vi "2D_Data_to_Igor_with_Prefix.vi"(6 "Do Transfer":bool=TRUE, 8 "error in (no error)":errorcluster, 9 "Wave Name":string, 10 "Wave Prefix":string, 11 "Data":dbl[][](array[numeric]) format="%.2f") -> (0 "error out":errorcluster, 2 "Wave Prefix Through":string)   [LabVIEW 2010]
uses:
  <vilib>/Utility/file.llb/Write To Spreadsheet File (DBL).vi
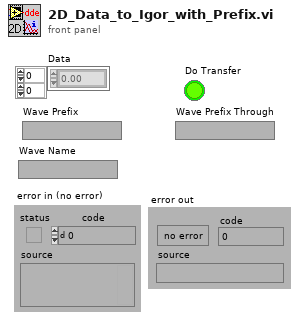
[diagram p1: front panel]
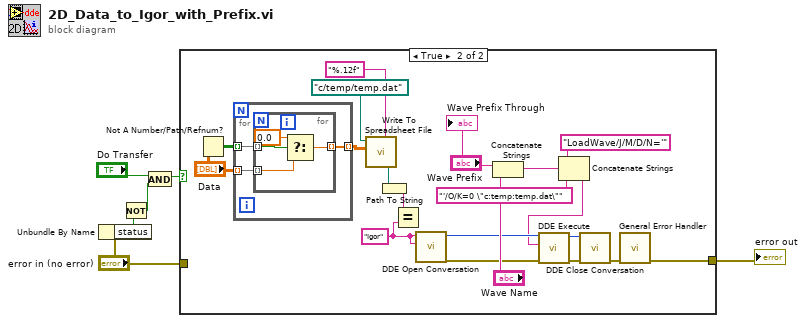
[diagram p0: block diagram]
diagram:
  n1 = Unbundle By Name("error in (no error)") -> ("status"=w4:bool)
  n2 = Not(x=w4) -> (.not. x?=w3:bool)
  n3 = And(x="Do Transfer", y=w3) -> (x .and. y?=w2:bool)
  n4 = case shown="True" w2 {
    tunnel: [w7 w25] -> w6
    tunnel: "error in (no error)" -> [w7 _]
    frame False {
    }
    frame True {
      w11 = "Igor" ("service")
      n5 = Not A Number/Path/Refnum?(number/path/refnum="Data") -> (NaN/Path/Refnum?=w26:bool[][])
      n6 = for {
        tunnel: w26 -> [w30] mode=indexing
        tunnel: "Data" -> [w29] mode=indexing
        tunnel: [w28] -> w13 mode=indexing
        n7 = for {
          tunnel: w30 -> [w34] mode=indexing
          tunnel: w29 -> [w33] mode=indexing
          tunnel: [w31] -> w28 mode=indexing
          n8 = Select(t=0.0, s=w34, f=w33) -> (s? t:f=w31:dbl)
        }
      }
      n9 = call-poly <vilib>:"Write To Spreadsheet File.vi"("format (%.3f)"="%.12f", "2D data"=w13, "file path (dialog if empty)"=path "c:/temp/temp.dat" ("Path")) -> ("new file path (Not A Path if cancelled)"=w10:path)  [unwired: 5 in]
      n10 = Path To String(path=w10) -> (string=w9:string)
      n11 = Equal?(x=w9, y=w11) -> ()  [unwired: 1 out]
      n12 = call "DDE Open Conversation.vi"("topic"=w11, "service"=w11) -> ("error out"=w19:errorcluster, "conversation refnum"=w22:u32)  [unwired: 6 in]
      n13 = Concatenate Strings("Wave Prefix", "Wave Name") -> (w17:string)
      n14 = Concatenate Strings("LoadWave/J/M/D/N='" ("command"), w17, "'/O/K=0 \"c:temp:temp.dat\"" ("command")) -> (w16:string)
      n15 = call <vilib>:"DDE Execute.vi"("error in (no error)"=w19, "command"=w16, "conversation refnum in"=w22) -> ("error out"=w20:errorcluster, "conversation refnum out"=w21:u32)  [unwired: 5 in]
      n16 = call "DDE Close Conversation.vi"("error in (no error)"=w20, "conversation refnum"=w21) -> ("error out"=w27:errorcluster)  [unwired: 7 in]
      n17 = call <vilib>:"General Error Handler.vi"("error in (no error)"=w27) -> ("error out"=w25:errorcluster)  [unwired: 10 in, 4 out]
      "Wave Prefix Through" <- "Wave Prefix"
    }
  }
  "error out" <- w6
